vi "VoltageOutput Example.vi"() -> ()   [LabVIEW 2012, in "Phidget Voltage Output.lvlib"]
uses:
  <instrlib>/Phidgets/Phidget Voltage Output/Phidget Voltage Output.lvlib
  <instrlib>/Phidgets/Phidget Voltage Output/Public/VoltageOutputStart.vi
  <instrlib>/Phidgets/Phidget Voltage Output/Public/VoltageOutputClose.vi
  <instrlib>/Phidgets/Phidget Common/Phidget Common.lvlib
panel:
  in  "Enabled":bool=TRUE
  in  "STOP":bool
  in  "Voltage Output Range":i32(ring)=1 items=["VOLTAGE_OUTPUT_RANGE_10V"=1, "VOLTAGE_OUTPUT_RANGE_5V"=2]
  in  "Voltage":dbl
  in  "error in (no error)":errorcluster
  in  "Device Info":T1={"Serial Number"=-1, "Channel"=0, "Port"=0}
  out "Attached?":bool
  out "error out":errorcluster
  # "Selecting Voltage Output Range is only \nnecessary for OUT1001 and OUT1002"
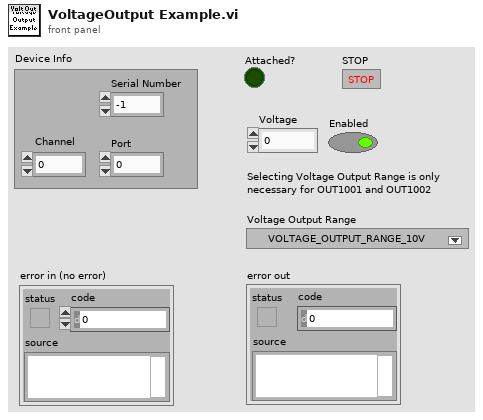
[diagram p1: front panel]
types:
  T1 = cluster{"Serial Number":i32, "Channel":i32, "Port":i32}
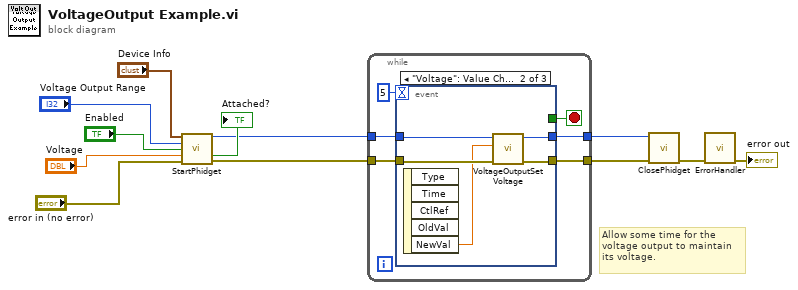
[diagram p0: block diagram]
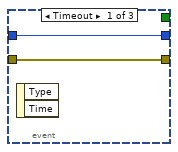
[diagram p2: hidden frame]
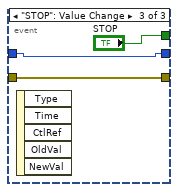
[diagram p3: hidden frame]
diagram:
  # "Allow some time for the\nvoltage output to maintain\nits voltage."
  n1 = call-poly <instrlib>:"StartPhidget.vi"("Device Info"="Device Info", "Voltage Output Range"="Voltage Output Range", "Enabled"="Enabled", "Voltage"="Voltage", "error in (no error)"="error in (no error)") -> ("Phidget ID"=w3:u64, "Attached?"=→"Attached?":bool, "error out"=w2:errorcluster)  [unwired: 7 in, 1 out]
  n2 = while {
    tunnel: w2 -> [w17]
    tunnel: w3 -> [w16]
    tunnel: [w15] -> w6
    tunnel: [w14] -> w7
    stop <- w13 stop-if-true
    n3 = event shown="[1] \"Voltage\": Value Change" {
      selector: _ -> [_ _ _]
      dyn-events: _ -> [_ _ _]
      timeout: 5 -> [_ _ _]
      tunnel: w16 -> [w20 w23 w27]
      tunnel: w17 -> [w19 w22 w26]
      tunnel: [w19 w25 w26] -> w14
      tunnel: [w20 w24 w27] -> w15
      tunnel: [_ _ "STOP"] -> w13
      event Timeout {
        n4 = event-data() -> ()  [unwired: 1 in, 2 out]
      }
      event "Voltage": Value Change {
        n5 = event-data() -> ("NewVal"=w21:dbl)  [unwired: 1 in, 4 out]
        n6 = call <instrlib>:"VoltageOutputSetVoltage.vi"("error in (no error)"=w22, "Voltage"=w21, "Device In"=w23) -> ("error out"=w25:errorcluster, "Device Out"=w24:u64)  [unwired: 6 in]
      }
      event "STOP": Value Change {
        n7 = event-data() -> ()  [unwired: 1 in, 5 out]
      }
    }
  }
  n8 = call-poly <instrlib>:"ClosePhidget.vi"("error in"=w7, "Device In"=w6) -> ("error out"=w12:errorcluster)  [unwired: 9 in]
  n9 = call <instrlib>:"ErrorHandler.vi"("error in"=w12) -> ("error out"=→"error out":errorcluster)  [unwired: 9 in, 1 out]
